vi "Select Group.vi"(8 "error in (no error)":errorcluster, 10 "Group":string, 11 "BluelinesRedlines in":refnum<class "BluelinesRedlines.lvclass">) -> (0 "error out":errorcluster, 3 "BluelinesRedlines out":refnum<class "BluelinesRedlines.lvclass">)   [LabVIEW 2020, in "VolatusGUIElements.lvlib" / "BluelinesRedlines.lvclass"]
uses:
  BluelinesRedlines.lvclass
  BluelinesRedlines.lvclass/BluelinesRedlines.ctl
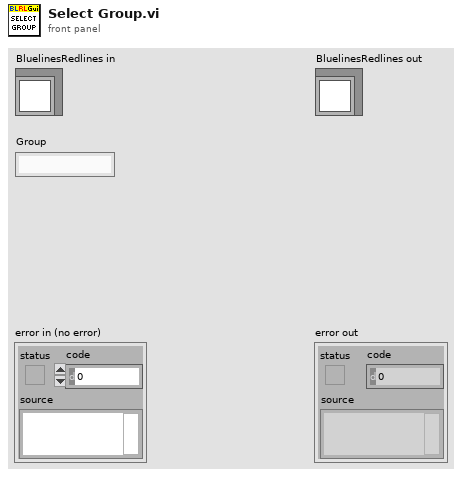
[diagram p1: front panel]
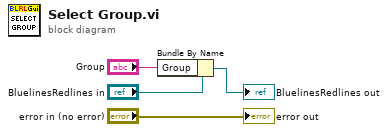
[diagram p0: block diagram]
diagram:
  n1 = Bundle By Name(cluster="BluelinesRedlines in", "Group"="Group") -> (→"BluelinesRedlines out":refnum<class "BluelinesRedlines.lvclass">)
  "error out" <- "error in (no error)"
